vi "PL_estimator.vi"(10 "initial parameters":dbl[](array[numeric])=[1.0, 1.0, 1.0, 1.0, 1.0], 11 "measured_signal":T1) -> (0 "quality_check":bool, 2 "fit_parameters":T3 {"mse" format="%#_3e"; "T1" format="%.3g"; "C1" format="%.3g"; "Tm" format="%.3g"; "Cm" format="%.3g"; "Ie" format="%.3g"}, 3 "fitted_signal":T2)   [LabVIEW 2018]
uses:
  <vilib>/Analysis/6fits.llb/Curve Fitting Criteria.ctl
  <vilib>/gmath/NumericalOptimization/Nonlinear Curve Fit LM bound.vi
  <vilib>/gmath/NI_Gmath.lvlib
  <vilib>/Analysis/NI_AALPro.lvlib
panel:
  in  "parameter maximum":dbl[](array[numeric])=[10.0, 0.9, 10.0, 10000.0]
  in  "parameter minimum":dbl[](array[numeric])=[1.0, 0.0001, 0.001, 10.0]
  out "XY Graph":T4(graph)
  # "Photoluminescence signal model:"
  # "I(t) = I(inf) * [1 - Cm * exp(-t/Tm) + C1 * exp(-t/T1)]"
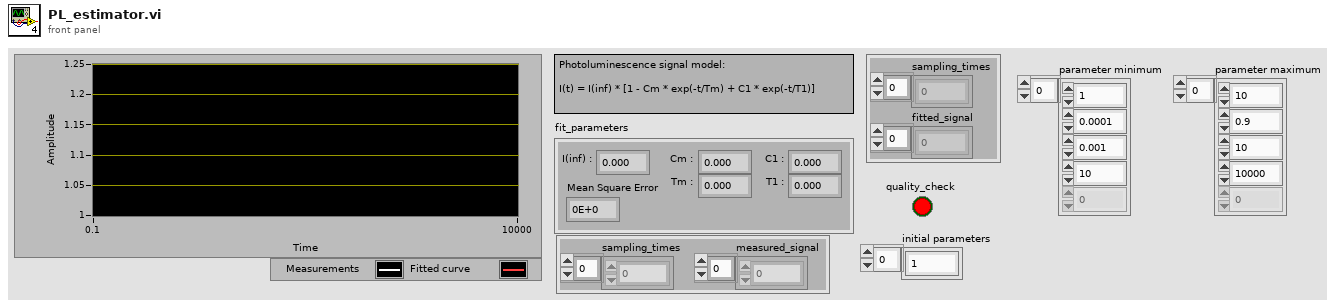
[diagram p1: front panel]
types:
  T1 = cluster{"sampling_times":dbl[], "measured_signal":dbl[]}
  T2 = cluster{"sampling_times":dbl[], "fitted_signal":dbl[]}
  T3 = cluster{"Ie":dbl, "Cm":dbl, "Tm":dbl, "C1":dbl, "T1":dbl, "mse":dbl}
  T4 = cluster{"log_samples_us":dbl[], "best nonlinear fit":dbl[]}[]
  T5 = cluster{"parameter minimum":dbl[], "parameter maximum":dbl[]}
  T6 = typedef "NI_AALPro.lvlib/Curve Fitting Criteria.ctl" = u16
  T7 = cluster{"sampling_times":dbl[], "best nonlinear fit":dbl[]}
  T8 = cluster{"sampling_times":dbl[], "best nonlinear fit":dbl[]}[]
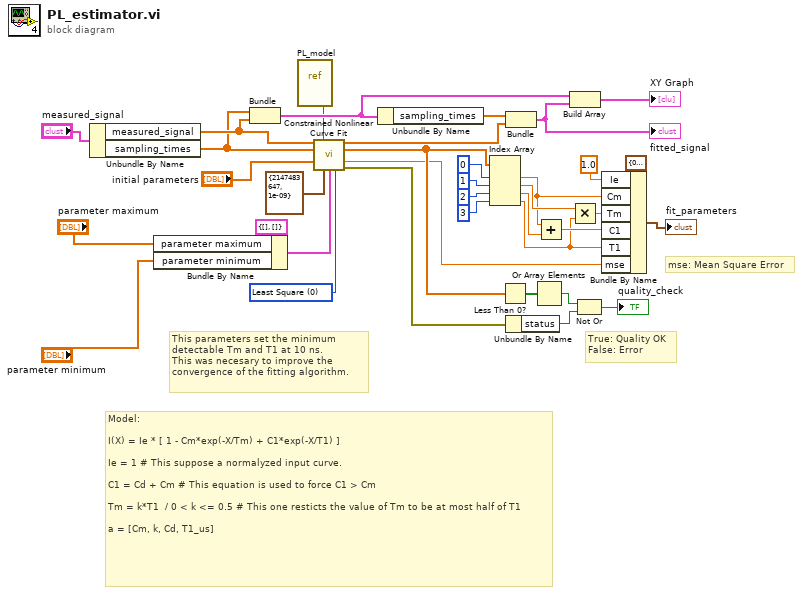
[diagram p0: block diagram]
diagram:
  w13 = T6 0 items=["Least Square", "Least Absolute Residual", "Bisquare"] ("method")
  # "Model:\n\nI(X) = Ie * [ 1 - Cm*exp(-X/Tm) + C1*exp(-X/T1) ]\n\nIe = 1 # This suppose a normalyzed input curve.\n\nC1 = Cd + Cm # This equation is used to force C1 > Cm\n\nTm = k*T1  / 0 < k <= 0.5 # This one resticts the value of Tm to be at most half of T1\n\na = [Cm, k, Cd, T1_us]"
  # "This parameters set the minimum \ndetectable Tm and T1 at 10 ns.\nThis was necesary to improve the\nconvergence of the fitting algorithm."
  # "True: Quality OK\nFalse: Error"
  # "mse: Mean Square Error"
  n1 = Unbundle By Name("measured_signal") -> ("measured_signal"=w23:dbl[], "sampling_times"=w22:dbl[])
  n2 = Bundle By Name(cluster=T5 {"parameter minimum"=[], "parameter maximum"=[]} ("parameter bounds"), "parameter maximum"="parameter maximum", "parameter minimum"="parameter minimum") -> (w8:T5)
  n3 = Bundle("sampling_times"=w22, "measured_signal"=w23) -> (w31:T1)  [unwired: 1 in]
  n4 = vi-ref "PL_model.vi"() -> (w18:refnum<vi>)
  n5 = call-poly <vilib>:"Constrained Nonlinear Curve Fit.vi"("Y"=w23, "f(x,a)"=w18, "X"=w22, "initial parameters"="initial parameters", "termination"=cluster{"max iteration":i32, "tolerance":dbl} {"max iteration"=2147483647, "tolerance"=1e-09}, "parameter bounds"=w8, "method"=w13) -> ("best nonlinear fit"=w19:dbl[], "best fit parameters"=w20:dbl[], "residue"=w14:dbl, "error out"=w21:errorcluster)  [unwired: 3 in, 2 out]
  n6 = Unbundle By Name(w31) -> ("sampling_times"=w29:dbl[])
  n7 = Index Array(array=w20, index #1=0 ("index"), index #2=1 ("index"), index #3=2 ("index"), index #4=3 ("index")) -> (element #1=w4:dbl, element #2=w6:dbl, element #3=w5:dbl, element #4=w1:dbl)
  n8 = Less Than 0?(x=w20) -> (x < 0?=w27:bool[])
  n9 = Bundle("sampling_times"=w29, "best nonlinear fit"=w19) -> (w36:T7)  [unwired: 1 in]
  "fitted_signal" <- w36
  n10 = Unbundle By Name(w21) -> ("status"=w25:bool)
  n11 = Or Array Elements(Boolean array=w27) -> (logical OR=w26:bool)
  n12 = Add(x=w4, y=w5) -> (x+y=w3:dbl)
  n13 = Build Array(w31, w36) -> (→"XY Graph":T8)
  n14 = Multiply(x=w6, y=w1) -> (x*y=w2:dbl)
  n15 = Not Or(1:w25, 2:w26) -> (0:→"quality_check":bool)
  n16 = Bundle By Name(cluster=T3 {"Ie"=0.0, "Cm"=0.0, "Tm"=0.0, "C1"=0.0, "T1"=0.0, "mse"=0.0} ("fit_parameters"), "Ie"=1.0, "Cm"=w4, "Tm"=w2, "C1"=w3, "T1"=w1, "mse"=w14) -> (→"fit_parameters":T3)
